vi "LoadModel.vi"(8 "error in (no error)":errorcluster, 10 "Actor In":refnum<class "Actor.lvclass">, 11 "GRMActor in":refnum<class "GenericController.lvclass">) -> (0 "error out":errorcluster, 3 "GRMActor out":refnum<class "GenericController.lvclass">)   [LabVIEW 2020, in "GenericController.lvlib" / "GenericController.lvclass"]
uses:
  GenericController.lvclass
  C:/Program Files/National Instruments/LabVIEW 2020/vi.lib/ActorFramework/Actor/Actor.lvclass
  <vilib>/ActorFramework/Actor/Actor.lvclass
  GenericController.lvclass/GenericController.ctl
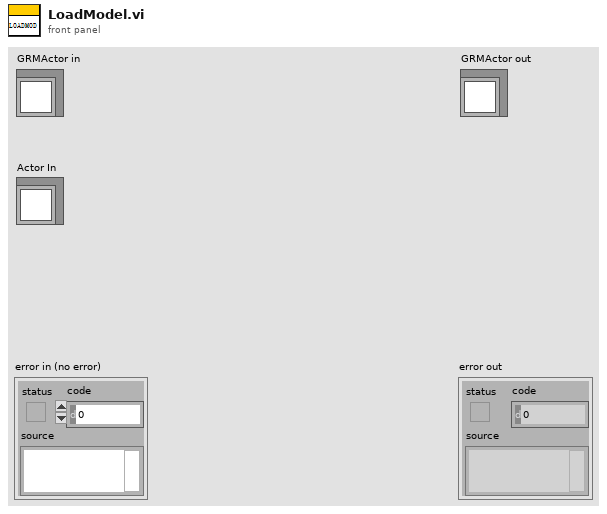
[diagram p1: front panel]
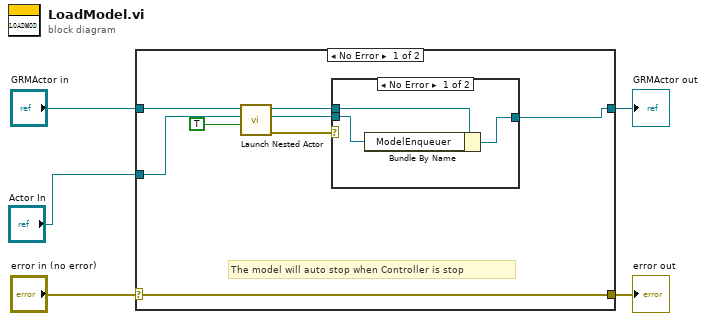
[diagram p0: block diagram]
diagram:
  n1 = case shown="No Error" "error in (no error)" {
    selector: "error in (no error)" -> [w13 w19]
    tunnel: [w13 w19] -> w4
    tunnel: [w9 w18] -> w2
    tunnel: "GRMActor in" -> [w11 w18]
    tunnel: "Actor In" -> [w12 _]
    frame No Error {
      # "The model will auto stop when Controller is stop"
      n2 = call <vilib>:"Launch Nested Actor.vi"("Auto-stop? (T)"=TRUE, "Nested Actor"=w12, "Caller Actor in"=w11) -> ("error out"=w7:errorcluster, "Nested Actor's Enqueuer"=w8:refnum<class "Message Enqueuer.lvclass">, "Caller Actor out"=w10:refnum<class "GenericController.lvclass">)  [unwired: 6 in]
      n3 = case shown="No Error" w7 {
        tunnel: w10 -> [w16 w17]
        tunnel: [w15 w17] -> w9
        tunnel: w8 -> [w14 _]
        frame No Error {
          n4 = Bundle By Name(cluster=w16, "ModelEnqueuer"=w14) -> (w15:refnum<class "GenericController.lvclass">)
        }
        frame Error {
        }
      }
    }
    frame Error {
    }
  }
  "error out" <- w4
  "GRMActor out" <- w2
